vi "freqAndNote.vi"() -> ()   [LabVIEW 2012]
uses:
  <vilib>/Utility/file.llb/Read From Spreadsheet File (string).vi
panel:
  out "Note Frequency":dbl
  in  "dt Original":dbl
  in  "Frequency In":dbl
  out "output dt":dbl
  out "Frequency Off":dbl
  out "Note Closest To":string
  # "This will pull out frequency difference and note and generate a dt to change frequency of signal.\nFirst generate note cluster array..."
  # "still fixing dt part I think it works though"
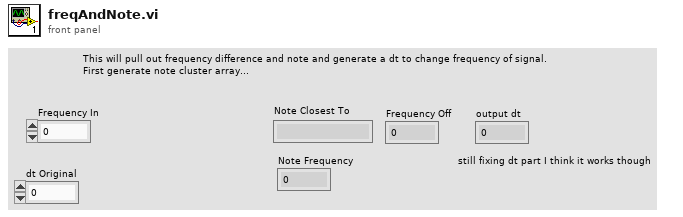
[diagram p1: front panel]
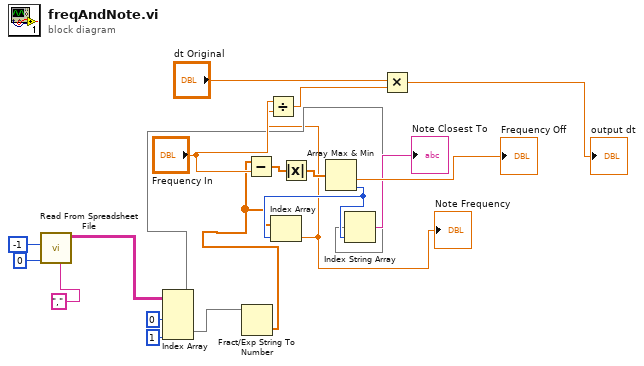
[diagram p0: block diagram]
diagram:
  n1 = call-poly <vilib>:"Read From Spreadsheet File.vi"("delimiter (\\t)"=",", "max characters/row  (no limit:0)"=0, "number of rows (all:-1)"=-1) -> ("all rows"=w8:string[][])  [unwired: 4 in, 4 out]
  n2 = Index Array(array=w8, index (col) #1=0 ("disabled index (col)"), index (col) #2=1 ("index (col)")) -> (element #1=w3:string[], element #2=w5:string[])  [unwired: 2 in]
  n3 = Fract/Exp String To Number(string=w5) -> (number=w4:dbl[])  [unwired: 3 in, 1 out]
  n4 = Subtract(x=w4, y="Frequency In") -> (x-y=w19:dbl[])
  n5 = Absolute Value(x=w19) -> (abs(x)=w18:dbl[])
  n6 = Array Max & Min(array=w18) -> (min value=→"Frequency Off":dbl, min index (indices)=w14:i32)  [unwired: 2 out]
  n7 = Index Array(array=w4, index=w14) -> (element=w1:dbl)
  "Note Frequency" <- w1
  n8 = Divide(x="Frequency In", y=w1) -> (x/y=w12:dbl)
  n9 = Index String Array(1:w14, 2:w3) -> (0:→"Note Closest To":string)  [unwired: 1 in]
  n10 = Multiply(x="dt Original", y=w12) -> (x*y=→"output dt":dbl)
